vi "Save vehicle navigation data in kml.vi"() -> ()   [LabVIEW 2015, in "Biblioteka moduł map v3.lvlib" / "KML.lvlib"]
uses:
  KML.lvlib
  KML point information.ctl
panel:
  in  "KML file":path
  out "text":string
  in  "file path (use dialog)":path
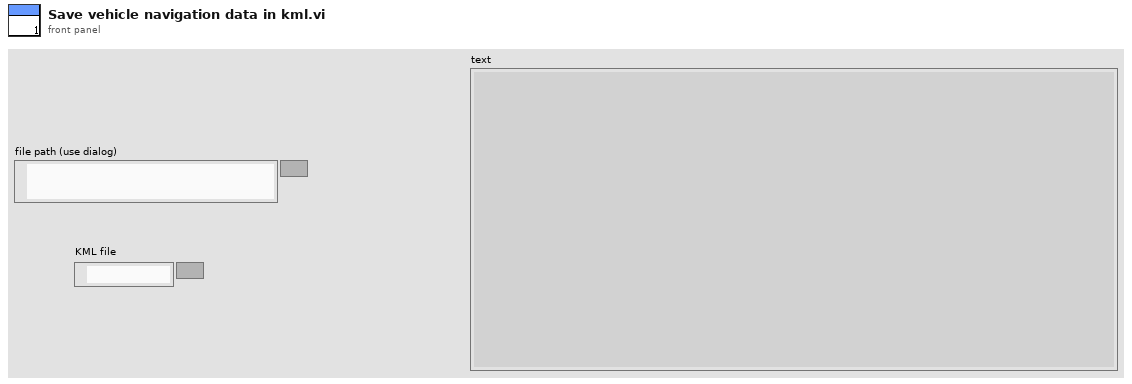
[diagram p1: front panel]
types:
  T1 = cluster{"Longitude":dbl, "Latitude":dbl, "Altitude":dbl}
  T2 = typedef "Biblioteka moduł map v3.lvlib/KML.lvlib/KML point information.ctl" = cluster{"Time UTC":string, "Heading":string, "Name path/point":string, "description":string}
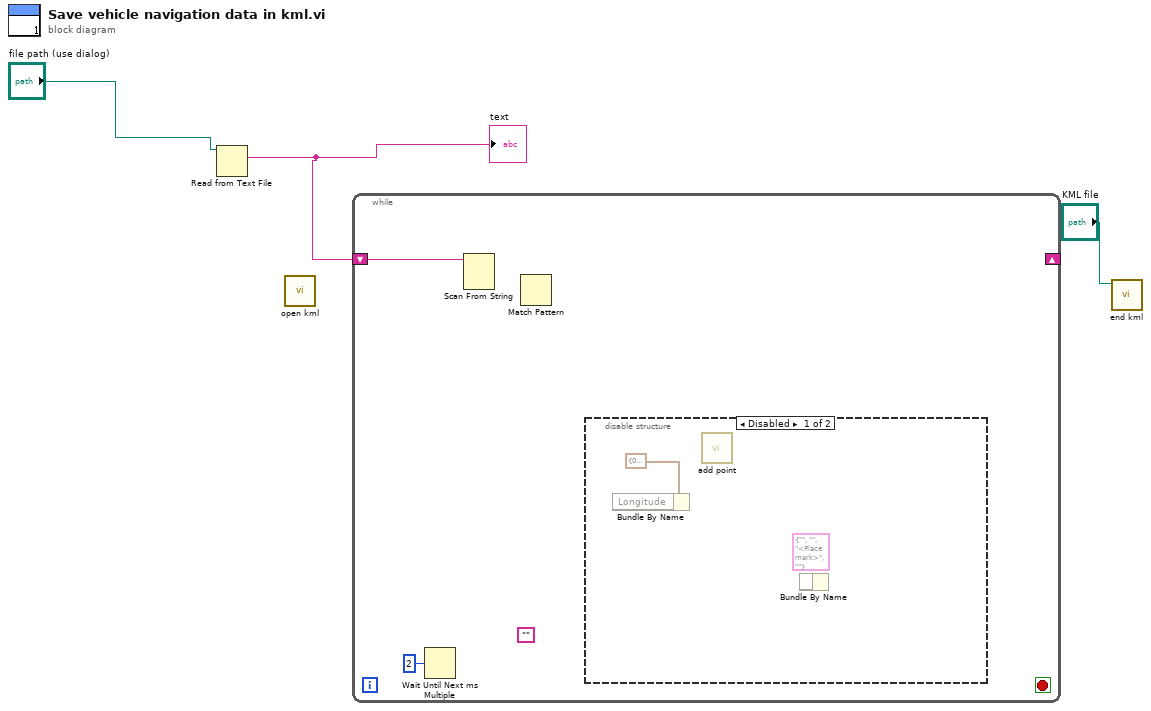
[diagram p0: block diagram]
diagram:
  n1 = Read from Text File(file (use dialog)="file path (use dialog)") -> (text=w2:string)  [unwired: 3 in, 3 out]
  "text" <- w2
  n2 = call "open kml.vi"() -> ()  [unwired: 5 in, 1 out]
  n3 = while {
    shift-right: _ -> [_]
    shift-left: w2 -> [w4]
    stop <- _ stop-if-true
    (unwired) ""
    n4 = Wait Until Next ms Multiple(millisecond multiple=u32 2) -> ()  [unwired: 1 out]
    n5 = Scan From String(input string=w4) -> ()  [unwired: 5 in, 3 out]
    n6 = Match Pattern() -> ()  [unwired: 3 in, 4 out]
    n7 = disable-structure shown="Disabled" {
      frame Disabled {
        (unwired) T2 {"Time UTC"="", "Heading"="", "Name path/point"="<Placemark>", "description"=""} ("Point information")
        n8 = Bundle By Name(cluster=T1 {"Longitude"=0.0, "Latitude"=0.0, "Altitude"=0.0} ("coordinates")) -> ()  [unwired: 1 in, 1 out]
        n9 = call "add point.vi"() -> ()  [unwired: 10 in, 1 out]
        n10 = Bundle By Name() -> ()  [unwired: 2 in, 1 out]
      }
      frame Enabled {
      }
    }
  }
  n11 = call "end kml.vi"("Path"="KML file") -> ()  [unwired: 7 in]
